vi "Periodic Tasks.vi"(8 "error in":errorcluster) -> ()   [LabVIEW 2014]
doc: "This VI runs in parallel to other tasks. It can contain as many user-defined periodic loops as you need. These can carry out PID or other sorts of timed response."
uses:
  Robot Global Data.vi
  <vilib>/Rock Robotics/Network Tables/SD Write Number.vi
  <vilib>/Rock Robotics/Network Tables/SD Write Boolean.vi
panel:
  out "Number Totes":dbl
  out "Autostacking":bool
  out "Up/Down Finished":bool
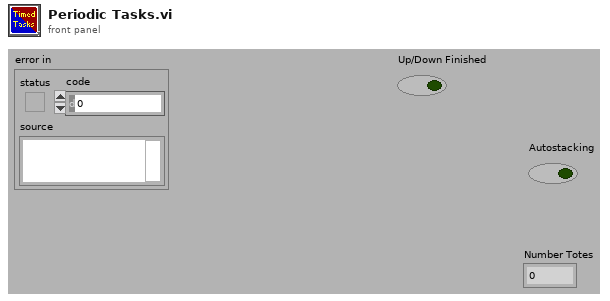
[diagram p1: front panel]
types:
  T1 = typedef "WPI_SwitchDevRef.ctl" = cluster{"DevStatus":errorcluster, "DIO Channel":T2, "Controller":T3, "CntIndex":T4, "Normally Closed":bool}
  T2 = typedef "FPGA_DIOChannel.ctl" = enum8{"DIO 0", "DIO 1", "DIO 2", "DIO 3", "DIO 4", "DIO 5", "DIO 6", "DIO 7", "DIO 8", "DIO 9", "DIO MXP 0", "DIO MXP 1", "DIO MXP 2", "DIO MXP 3", "DIO MXP 4", "DIO MXP 5", "DIO MXP 6", "DIO MXP 7", "DIO MXP 8", "DIO MXP 9", "DIO MXP 10", "DIO MXP 11", "DIO MXP 12", "DIO MXP 13", "DIO MXP 14", "DIO MXP 15", "Invalid"}
  T3 = typedef "FPGA_TypedefDigitalModule.ctl" = enum16{"Controller 1"}
  T4 = typedef "FPGA_CounterCtrSystemIndex.ctl" = enum8{"Ctr 0", "Ctr 1", "Ctr 2", "Ctr 3", "Ctr 4", "Ctr 5", "Ctr 6", "Ctr 7", "Invalid"}
  T5 = typedef "WPI_EncoderDevRef.ctl" = cluster{"DevStatus":errorcluster, "EncoderIndex":T6, "CounterIndex":T4, "DistancePerCount":dbl, "Decoding Type":T7}
  T6 = typedef "FPGA_EncoderIdx.ctl" = enum8{"Enc 0", "Enc 1", "Enc 2", "Enc 3", "Enc 4", "Enc 5", "Enc 6", "Enc 7", "Invalid"}
  T7 = typedef "WPI_EncoderType.ctl" = enum16{"1x", "2x", "4x"}
  T8 = typedef "WPI_PotentiometerDevRef.ctl" = cluster{"DevStatus":errorcluster, "Controller":T9, "Analog Channel":T10, "Invert Output":bool}
  T9 = typedef "FPGA_TypedefAnalogModule.ctl" = enum16{"Controller 1"}
  T10 = typedef "FPGA_AIChannel.ctl" = enum8{"AI 0", "AI 1", "AI 2", "AI 3", "AI MXP 0", "AI MXP 1", "AI MXP 2", "AI MXP 3", "Invalid"}
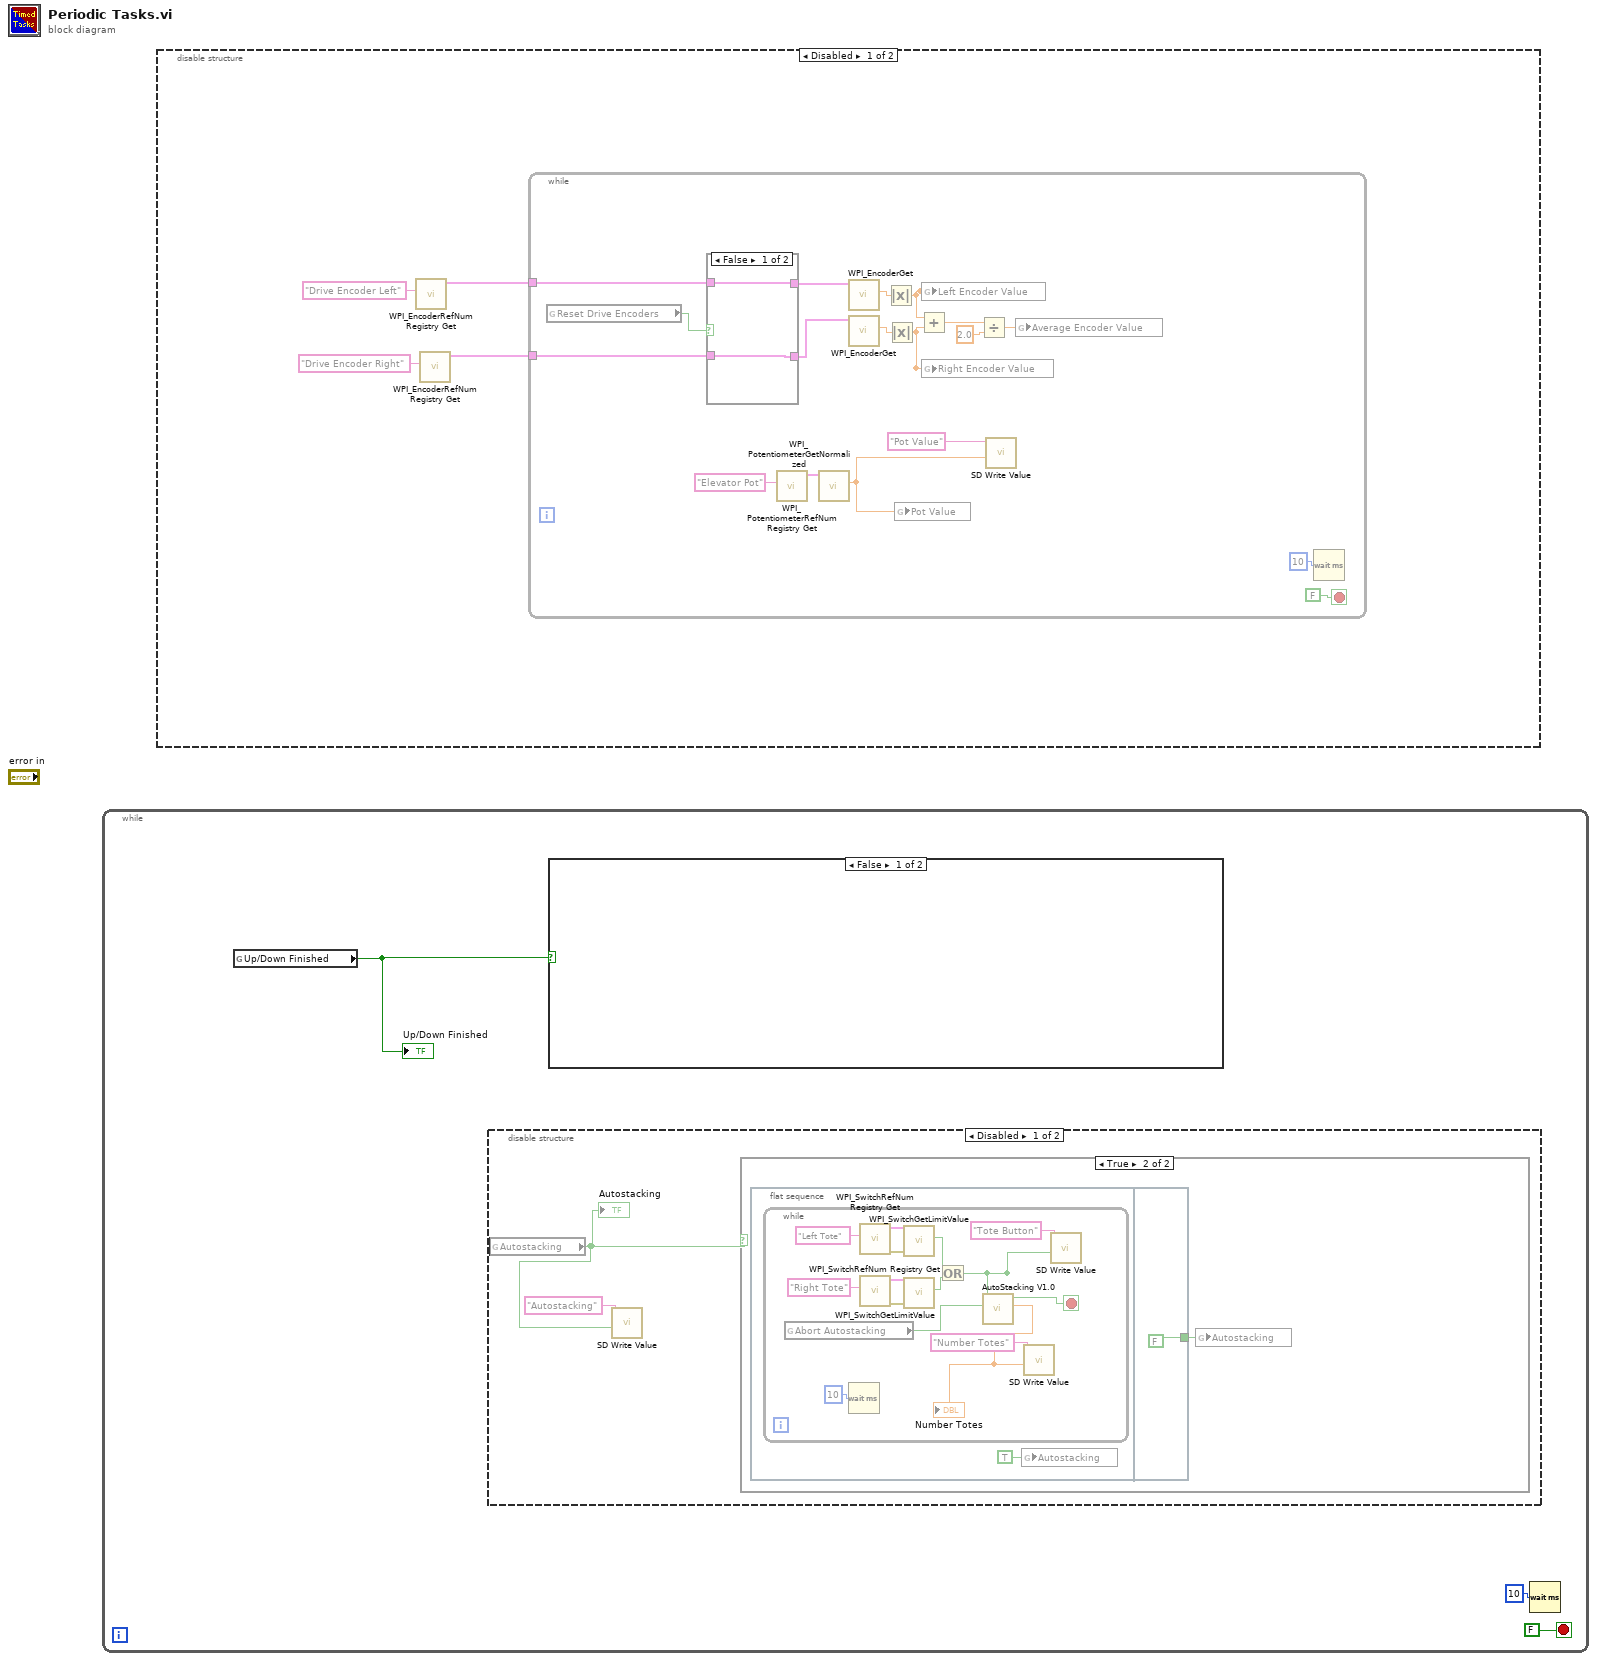
[diagram p0: block diagram]
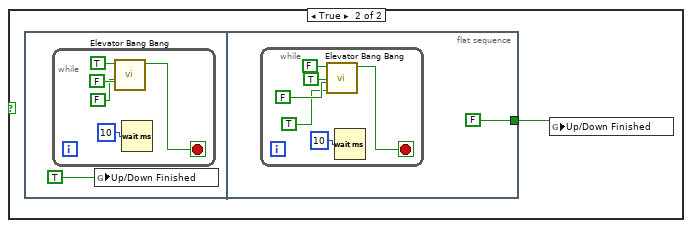
[diagram p4: hidden frame]
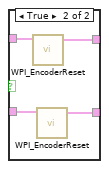
[diagram p5: hidden frame]
diagram:
  n1 = while {
    stop <- FALSE stop-if-true
    n2 = global read "Robot Global Data.vi" "Up/Down Finished"() -> (w1:bool)
    "Up/Down Finished" <- w1
    n3 = disable-structure shown="Disabled" {
      frame Disabled {
        n4 = global read "Robot Global Data.vi" "Autostacking"() -> (w4:bool)
        "Autostacking" <- w4
        n5 = call-poly <vilib>:"SD Write Value.vi"("Boolean"=w4, "Name"="Autostacking") -> ()  [unwired: 8 in, 2 out]
        n6 = case shown="True" w4 {
          frame False {
          }
          frame True {
            n7 = flat-sequence {
              tunnel: [FALSE] -> w6
              frame #0 {
                n8 = while {
                  stop <- w22 stop-if-true
                  n9 = global read "Robot Global Data.vi" "Abort Autostacking"() -> (w20:bool)
                  n10 = Wait (ms)(milliseconds to wait=u32 10) -> ()  [unwired: 1 out]
                  n11 = call <vilib>:"WPI_SwitchRefNum Registry Get.vi"("refnum name"="Left Tote") -> ("error out"=w12:errorcluster, "SwitchDevRef"=w13:T1)  [unwired: 9 in]
                  n12 = call <vilib>:"WPI_SwitchRefNum Registry Get.vi"("refnum name"="Right Tote") -> ("error out"=w17:errorcluster, "SwitchDevRef"=w16:T1)  [unwired: 9 in]
                  n13 = call <vilib>:"WPI_SwitchGetLimitValue.vi"("error in (no error)"=w12, "SwitchDevRef"=w13) -> ("Switch Pressed"=w18:bool)  [unwired: 7 in, 2 out]
                  n14 = call <vilib>:"WPI_SwitchGetLimitValue.vi"("error in (no error)"=w17, "SwitchDevRef"=w16) -> ("Switch Pressed"=w19:bool)  [unwired: 7 in, 2 out]
                  n15 = Or(x=w18, y=w19) -> (x .or. y?=w8:bool)
                  n16 = call "AutoStacking V1.0.vi"("Abort"=w20, "Tote Button"=w8) -> ("Number Totes"=w11:dbl, "Finished"=w22:bool)  [unwired: 8 in]
                  "Number Totes" <- w11
                  n17 = call-poly <vilib>:"SD Write Value.vi"("Numeric"=w11, "Name"="Number Totes") -> ()  [unwired: 8 in, 2 out]
                  n18 = call-poly <vilib>:"SD Write Value.vi"("Boolean"=w8, "Name"="Tote Button") -> ()  [unwired: 8 in, 2 out]
                }
                n19 = global write "Robot Global Data.vi" "Autostacking"(TRUE ("Autostacking")) -> ()
              }
              frame #1 {
              }
            }
            n20 = global write "Robot Global Data.vi" "Autostacking"(w6) -> ()
          }
        }
      }
      frame Enabled {
      }
    }
    n21 = case shown="False" w1 {
      frame False {
      }
      frame True {
        n22 = flat-sequence {
          tunnel: [FALSE ("Button 3")] -> w24
          frame #0 {
            n23 = while {
              stop <- w27 stop-if-true
              n24 = call "Elevator Bang Bang.vi"("Top"=FALSE ("Button 3"), "Middle"=FALSE ("Button 2"), "Bottom"=TRUE ("Button 1")) -> ("in range"=w27:bool)  [unwired: 8 in]
              n25 = Wait (ms)(milliseconds to wait=u32 10) -> ()  [unwired: 1 out]
            }
            n26 = global write "Robot Global Data.vi" "Up/Down Finished"(TRUE ("Button 3")) -> ()
          }
          frame #1 {
            n27 = while {
              stop <- w34 stop-if-true
              n28 = call "Elevator Bang Bang.vi"("Hold Up Mode"=TRUE, "Top"=FALSE ("Button 3"), "Middle"=TRUE ("Button 2"), "Bottom"=FALSE ("Button 1")) -> ("in range"=w34:bool)  [unwired: 7 in]
              n29 = Wait (ms)(milliseconds to wait=u32 10) -> ()  [unwired: 1 out]
            }
          }
        }
        n30 = global write "Robot Global Data.vi" "Up/Down Finished"(w24) -> ()
      }
    }
    n31 = Wait (ms)(milliseconds to wait=u32 10) -> ()  [unwired: 1 out]
  }
  n32 = disable-structure shown="Disabled" {
    frame Disabled {
      n33 = call <vilib>:"WPI_EncoderRefNum Registry Get.vi"("refnum name"="Drive Encoder Left") -> ("EncoderDevRef"=w41:T5)  [unwired: 9 in, 1 out]
      n34 = call <vilib>:"WPI_EncoderRefNum Registry Get.vi"("refnum name"="Drive Encoder Right") -> ("EncoderDevRef"=w40:T5)  [unwired: 9 in, 1 out]
      n35 = while {
        tunnel: w41 -> [w57]
        tunnel: w40 -> [w53]
        stop <- FALSE stop-if-true
        n36 = global read "Robot Global Data.vi" "Reset Drive Encoders"() -> (w55:bool)
        n37 = case shown="False" w55 {
          tunnel: w57 -> [w60 w65]
          tunnel: [w60 w64] -> w56
          tunnel: w53 -> [w61 w62]
          tunnel: [w61 w63] -> w54
          frame False {
          }
          frame True {
            n38 = call <vilib>:"WPI_EncoderReset.vi"("EncoderDevRef"=w65) -> ("EncoderDevRef"=w64:T5)  [unwired: 9 in, 1 out]
            n39 = call <vilib>:"WPI_EncoderReset.vi"("EncoderDevRef"=w62) -> ("EncoderDevRef"=w63:T5)  [unwired: 9 in, 1 out]
          }
        }
        n40 = call <vilib>:"WPI_PotentiometerRefNum Registry Get.vi"("refnum name"="Elevator Pot") -> ("PotDevRef"=w50:T8)  [unwired: 9 in, 1 out]
        n41 = call <vilib>:"WPI_PotentiometerGetNormalized.vi"("PotDevRef"=w50) -> ("Normalized Value"=w48:dbl)  [unwired: 8 in, 2 out]
        n42 = call <vilib>:"WPI_EncoderGet.vi"("EncoderDevRef"=w56) -> ("Distance"=w43:dbl)  [unwired: 5 in, 5 out]
        n43 = call <vilib>:"WPI_EncoderGet.vi"("EncoderDevRef"=w54) -> ("Distance"=w45:dbl)  [unwired: 5 in, 5 out]
        n44 = Absolute Value(x=w43) -> (abs(x)=w42:dbl)
        n45 = Absolute Value(x=w45) -> (abs(x)=w44:dbl)
        n46 = global write "Robot Global Data.vi" "Pot Value"(w48) -> ()
        n47 = Add(x=w42, y=w44) -> (x+y=w52:dbl)
        n48 = global write "Robot Global Data.vi" "Left Encoder Value"(w42) -> ()
        n49 = global write "Robot Global Data.vi" "Right Encoder Value"(w44) -> ()
        n50 = Divide(x=w52, y=2.0) -> (x/y=w46:dbl)
        n51 = call-poly <vilib>:"SD Write Value.vi"("Numeric"=w48, "Name"="Pot Value") -> ()  [unwired: 8 in, 2 out]
        n52 = global write "Robot Global Data.vi" "Average Encoder Value"(w46) -> ()
        n53 = Wait (ms)(milliseconds to wait=u32 10) -> ()  [unwired: 1 out]
      }
    }
    frame Enabled {
    }
  }
